vi "Request New Token with Login Credentials.vi"(8 "error in":errorcluster, 9 "expires in (s)":i32=-1, 10 "password":string, 11 "username":string) -> (0 "error out":errorcluster, 3 "token response":T1)   [LabVIEW 2013, in "Particle API.lvlib"]
uses:
  Particle API.lvlib
  Controls/Token Response JSON.ctl
  <vilib>/httpClient/POSTBuffer.vi
  <vilib>/httpClient/LabVIEWHTTPClient.lvlib
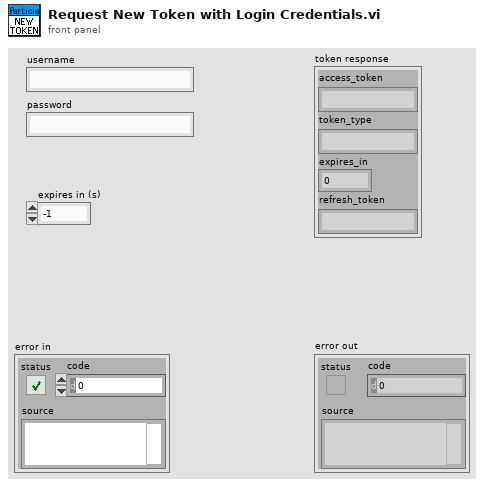
[diagram p1: front panel]
types:
  T1 = typedef "Particle API.lvlib/Token Response JSON.ctl" = cluster{"access_token":string, "token_type":string, "expires_in":dbl, "refresh_token":string}
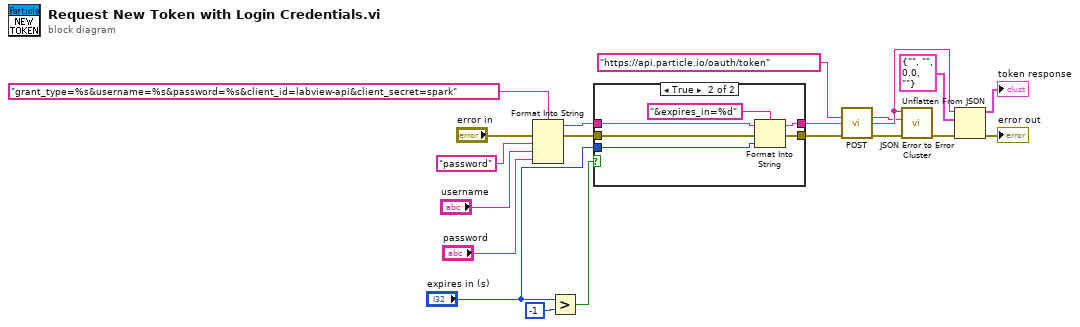
[diagram p0: block diagram]
diagram:
  n1 = Format Into String(format string="grant_type=%s&username=%s&password=%s&client_id=labview-api&client_secret=spark", error in="error in", "password" ("Grant Type"), "username", "password") -> (resulting string=w6:string, error out=w3:errorcluster)  [unwired: 1 in]
  n2 = Greater?(x="expires in (s)", y=-1) -> (0:w7:bool)
  n3 = case shown="True" w7 {
    tunnel: w6 -> [w22 w28]
    tunnel: "expires in (s)" -> [_ w26]
    tunnel: [w22 w25] -> w4
    tunnel: w3 -> [w21 w24]
    tunnel: [w21 w23] -> w2
    frame False {
    }
    frame True {
      n4 = Format Into String(format string="&expires_in=%d", initial string=w28, error in=w24, w26) -> (resulting string=w25:string, error out=w23:errorcluster)
    }
  }
  n5 = call-poly <vilib>:"POST.vi"("url"="https://api.particle.io/oauth/token", "buffer"=w4, "error in (no error)"=w2) -> ("headers"=w11:string, "body"=w12:string, "error out"=w15:errorcluster)  [unwired: 9 in, 1 out]
  n6 = call "JSON Error to Error Cluster.vi"("error in (no error)"=w15, "headers"=w11, "JSON string"=w12) -> ("error out"=w13:errorcluster)  [unwired: 8 in]
  n7 = Unflatten From JSON(JSON string=w12, type and defaults=T1 {"access_token"="", "token_type"="", "expires_in"=0.0, "refresh_token"=""} ("Function Response"), error in (no error)=w13) -> (value=→"token response":T1, error out=→"error out":errorcluster)  [unwired: 4 in]
